vi "Teleop.vi"(10 "Match Info":T1={"Autonomous Elapsed Seconds"=0.0, "TeleOp Elapsed Seconds"=0.0, "Disabled Elapsed Seconds"=0.0, "Visited Autonomous"=FALSE, "Visited TeleOp"=FALSE, "Visited Disabled"=FALSE, "Autonomous Settings"={"Autonomous Style"=enum."Independent", "VI Refnum"=refnum}}, 11 "Call Context":T2) -> ()   [LabVIEW 2016]
doc: "This VI is called for each TeleOp packet received from the DS where the robot is not disabled. It is often used to read from the joysticks and update I/O or to update setpoints for timed control loops. It should complete and return within 20 milliseconds or it may miss DS packets."
uses:
  <vilib>/Rock Robotics/WPI/DriverStation/WPI_DriverStationDerivedRobotMode.ctl
  <vilib>/Rock Robotics/WPI/DriverStation/WPI_DriverStationMatch Info.ctl
  <vilib>/Rock Robotics/WPI/Solenoid/WPI_SolenoidValue.ctl
  <vilib>/Rock Robotics/WPI/Utilities/WPI_GetSetVariantRefNum.vi
  <vilib>/Rock Robotics/Network Tables/NT Write Boolean Array.vi
  <vilib>/Rock Robotics/Network Tables/NT Write Numeric Array.vi
  <vilib>/Rock Robotics/Network Tables/NT Read Boolean.vi
  <vilib>/Rock Robotics/Network Tables/NT Read Number.vi
  <vilib>/Rock Robotics/WPI/Solenoid/WPI_SolenoidSetEnum.vi
  <vilib>/Rock Robotics/Network Tables/NT Write Boolean.vi
  <vilib>/Rock Robotics/WPI/RobotDrive/WPI_RobotDriveArcadeDrive_Standard(NoSaturation).vi
panel:
  out "Sample Slider 0":dbl(slide) scale=0.0..5.0
  out "Sample Boolean 1":bool
  out "Sample Boolean 0":bool
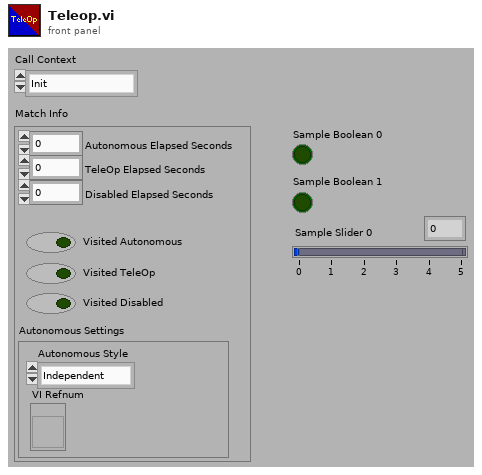
[diagram p1: front panel]
types:
  T1 = typedef "WPI_DriverStationMatch Info.ctl" = cluster{"Autonomous Elapsed Seconds":dbl, "TeleOp Elapsed Seconds":dbl, "Disabled Elapsed Seconds":dbl, "Visited Autonomous":bool, "Visited TeleOp":bool, "Visited Disabled":bool, "Autonomous Settings":cluster{"Autonomous Style":enum16{"Iterative", "Independent"}, "VI Refnum":refnum<vi>}}
  T2 = typedef "WPI_DriverStationDerivedRobotMode.ctl" = enum16{"Init", "Execute", "Stop"}
  T3 = typedef "WPI_SolenoidValue.ctl" = enum16{"Off", "On", "Forward", "Reverse"}
  T4 = typedef "WPI_MotorControlDeviceRef.ctl" = cluster{"DeviceStatus":errorcluster, "Type":T5, "PWM":cluster{"PWM Channel":T6, "DeadBand":T7}, "CAN":cluster{"Device Number":u8, "SetOutput VI Ref":variant, "GetOutput VI Ref":variant, "Enable VI Ref":variant, "Disable VI Ref":variant, "Data":variant}, "Invert":bool}
  T5 = typedef "WPI_MotorControlType.ctl" = enum16{"PWM", "CAN"}
  T6 = typedef "FPGA_DIOPWMChannel.ctl" = enum8{"PWM 0", "PWM 1", "PWM 2", "PWM 3", "PWM 4", "PWM 5", "PWM 6", "PWM 7", "PWM 8", "PWM 9", "PWM MXP 0", "PWM MXP 1", "PWM MXP 2", "PWM MXP 3", "PWM MXP 4", "PWM MXP 5", "PWM MXP 6", "PWM MXP 7", "PWM MXP 8", "PWM MXP 9", "Invalid"}
  T7 = typedef "WPI_PWMDeadband.ctl" = cluster{"Name":string, "maxPositivePwm":i32, "minPositivePwm":i32, "centerPwm":i32, "maxNegativePwm":i32, "minNegativePwm":i32, "angularRange":u16}
  T8 = typedef "WPI_RobotDriveDevRef.ctl" = cluster{"DevStatus":errorcluster, "Motors[]":T4[], "Square Inputs":bool, "Max Output":dbl}
  T9 = typedef "WPI_JoystickDevRef.ctl" = cluster{"Device":T10}
  T10 = typedef "WPI_JoystickDeviceEnum.ctl" = enum16{"USB 0", "USB 1", "USB 2", "USB 3", "USB 4", "USB 5"}
  T11 = typedef "WPI_SolenoidDevRef.ctl" = cluster{"DevStatus":errorcluster, "Pneumatics Control Module":u8, "Forward Solenoid Channel":T12, "Reverse Solenoid Channel":T12}
  T12 = typedef "WPI_SolenoidChannel.ctl" = enum8{"Solenoid 0", "Solenoid 1", "Solenoid 2", "Solenoid 3", "Solenoid 4", "Solenoid 5", "Solenoid 6", "Solenoid 7", "Invalid"}
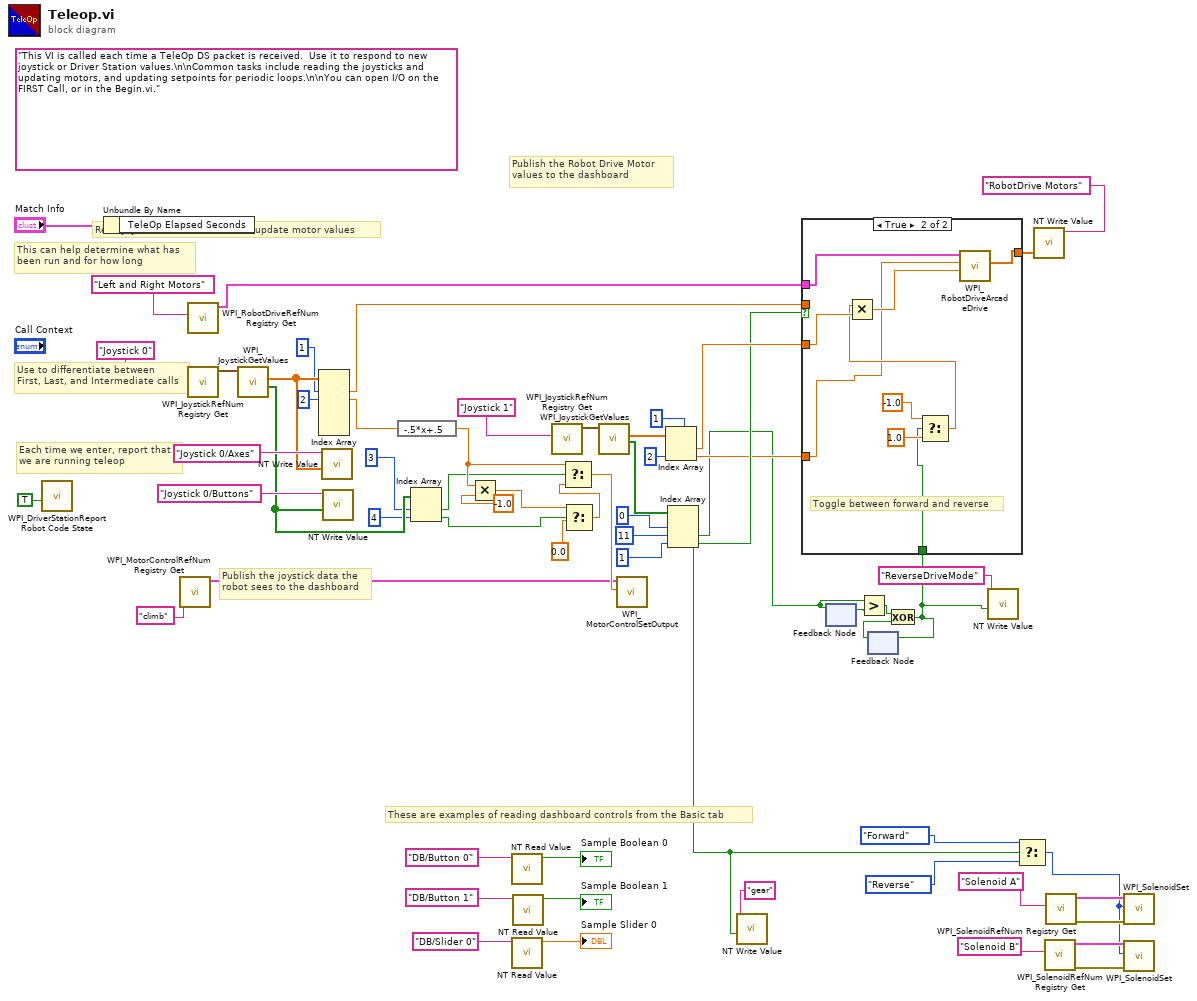
[diagram p0: block diagram]
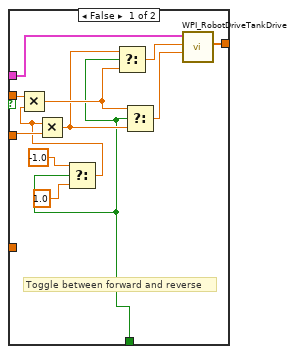
[diagram p2: hidden frame]
diagram:
  (unwired) "This VI is called each time a TeleOp DS packet is received.  Use it to respond to new joystick or Driver Station values.\n\nCommon tasks include reading the joysticks and updating motors, and updating setpoints for periodic loops.\n\nYou can open I/O on the FIRST Call, or in the Begin.vi."
  # "Publish the Robot Drive Motor\nvalues to the dashboard"
  # "These are examples of reading dashboard controls from the Basic tab"
  # "Publish the joystick data the\nrobot sees to the dashboard"
  # "Each time we enter, report that\nwe are running teleop"
  # "Use to differentiate between\nFirst, Last, and Intermediate calls"
  # "This can help determine what has\nbeen run and for how long"
  # "Read Joystick X and Y values and update motor values"
  n1 = call <vilib>:"WPI_DriverStationReport Robot Code State.vi"("TeleOp"=TRUE ("Autonomous")) -> ()  [unwired: 10 in, 1 out]
  n2 = Unbundle By Name("Match Info") -> ()  [unwired: 1 out]
  n3 = call <vilib>:"WPI_MotorControlRefNum Registry Get.vi"("refnum name"="climb") -> ("MotorControlDevRef"=w25:T4)  [unwired: 9 in, 1 out]
  n4 = call <vilib>:"WPI_RobotDriveRefNum Registry Get.vi"("refnum name"="Left and Right Motors") -> ("RobotDriveDevRef"=w20:T8)  [unwired: 1 in, 9 out]
  n5 = call <vilib>:"WPI_JoystickRefNum Registry Get.vi"("refnum name"="Joystick 0") -> ("JoystickDevRef"=w60:T9)  [unwired: 1 in, 9 out]
  n6 = call <vilib>:"WPI_JoystickGetValues.vi"("JoystickDevRef"=w60) -> ("Buttons"=w34:bool[], "Axes"=w56:dbl[])  [unwired: 6 in, 3 out]
  n7 = Index Array(array=w56, index #1=1 ("index"), index #2=2 ("index")) -> (element #1=w19:dbl, element #2=w31:dbl)  [unwired: 4 in, 4 out]
  n8 = call-poly <vilib>:"NT Write Value.vi"("Numeric Array"=w56, "Name"="Joystick 0/Axes") -> ()  [unwired: 9 in, 1 out]
  n9 = call-poly <vilib>:"NT Write Value.vi"("Boolean Array"=w34, "Name"="Joystick 0/Buttons") -> ()  [unwired: 9 in, 1 out]
  n10 = expression code="-.5*x+.5"(w31) -> (w30:dbl)
  n11 = Index Array(array=w34, index #1=3 ("index"), index #2=4 ("index")) -> (element #1=w21:bool, element #2=w22:bool)
  n12 = Multiply(x=w30, y=-1.0) -> (x*y=w27:dbl)
  n13 = call-poly <vilib>:"NT Read Value.vi"("Name"="DB/Button 0" ("refnum name")) -> ("Boolean"=→"Sample Boolean 0":bool)  [unwired: 9 in, 1 out]
  n14 = call-poly <vilib>:"NT Read Value.vi"("Name"="DB/Slider 0" ("refnum name")) -> ("Numeric"=→"Sample Slider 0":dbl)  [unwired: 9 in, 1 out]
  n15 = call-poly <vilib>:"NT Read Value.vi"("Name"="DB/Button 1" ("refnum name")) -> ("Boolean"=→"Sample Boolean 1":bool)  [unwired: 9 in, 1 out]
  n16 = call <vilib>:"WPI_JoystickRefNum Registry Get.vi"("refnum name"="Joystick 1") -> ("JoystickDevRef"=w38:T9)  [unwired: 1 in, 9 out]
  n17 = Select(t=w27, s=w22, f=0.0) -> (s? t:f=w23:dbl)
  n18 = Select(t=w30, s=w21, f=w23) -> (s? t:f=w28:dbl)
  n19 = call <vilib>:"WPI_JoystickGetValues.vi"("JoystickDevRef"=w38) -> ("Buttons"=w11:bool[], "Axes"=w37:dbl[])  [unwired: 6 in, 3 out]
  n20 = call <vilib>:"WPI_MotorControlSetOutput.vi"("Output"=w28, "MotorControlDevRef"=w25) -> ()  [unwired: 7 in, 3 out]
  n21 = Index Array(array=w37, index #1=1 ("index"), index #2=2 ("index")) -> (element #1=w18:dbl, element #2=w13:dbl)
  n22 = Index Array(array=w11, index #1=0 ("index"), index #2=11 ("index"), index #3=1 ("index")) -> (element #1=w8:bool, element #2=w3:bool, element #3=w14:bool)
  n23 = call-poly <vilib>:"NT Write Value.vi"("Boolean"=w8, "Name"="gear") -> ()  [unwired: 9 in, 1 out]
  n24 = feedback #1() -> (w5:bool)  [unwired: 1 in]
  n25 = feedback-in #1(w3) -> ()
  n26 = Greater?(x=w3, y=w5) -> (0:w4:bool)
  n27 = feedback #2() -> (w6:bool)  [unwired: 1 in]
  n28 = Exclusive Or(1:w6, 2:w4) -> (0:w2:bool)
  n29 = case shown="True" w14 {
    tunnel: w20 -> [w70 w83]
    tunnel: w19 -> [w73 _]
    tunnel: w18 -> [w71 w80]
    tunnel: [w72 w84] -> w16
    tunnel: w13 -> [_ w76]
    tunnel: w2 -> [w64 w77]
    frame False {
      # "Toggle between forward and reverse"
      n30 = Select(t=-1.0, s=w64, f=1.0) -> (s? t:f=w65:dbl)
      n31 = Multiply(x=w73, y=w65) -> (x*y=w68:dbl)
      n32 = Multiply(x=w65, y=w71) -> (x*y=w66:dbl)
      n33 = Select(t=w66, s=w64, f=w68) -> (s? t:f=w67:dbl)
      n34 = Select(t=w68, s=w64, f=w66) -> (s? t:f=w69:dbl)
      n35 = call <vilib>:"WPI_RobotDriveTankDrive.vi"("Right axis value"=w69, "Left axis value"=w67, "RobotDriveDevRef"=w70) -> ("Motor Values"=w72:dbl[])  [unwired: 6 in, 2 out]
    }
    frame True {
      # "Toggle between forward and reverse"
      n36 = Select(t=-1.0, s=w77, f=1.0) -> (s? t:f=w79:dbl)
      n37 = Multiply(x=w79, y=w80) -> (x*y=w78:dbl)
      n38 = call-poly <vilib>:"WPI_RobotDriveArcadeDrive.vi"("Y axis value"=w78, "X axis value"=w76, "RobotDriveDevRef"=w83) -> ("Motor Values"=w84:dbl[])  [unwired: 6 in, 2 out]
    }
  }
  n39 = feedback-in #2(w2) -> ()
  n40 = call-poly <vilib>:"NT Write Value.vi"("Boolean"=w2, "Name"="ReverseDriveMode") -> ()  [unwired: 9 in, 1 out]
  n41 = Select(t=WPI_SolenoidValue."Forward" ("Value"), s=w8, f=WPI_SolenoidValue."Reverse" ("Value")) -> (s? t:f=w40:T3)
  n42 = call-poly <vilib>:"NT Write Value.vi"("Numeric Array"=w16, "Name"="RobotDrive Motors") -> ()  [unwired: 9 in, 1 out]
  n43 = call <vilib>:"WPI_SolenoidRefNum Registry Get.vi"("refnum name"="Solenoid B") -> ("error out"=w42:errorcluster, "SolenoidDevRef"=w43:T11)  [unwired: 9 in]
  n44 = call <vilib>:"WPI_SolenoidRefNum Registry Get.vi"("refnum name"="Solenoid A") -> ("error out"=w47:errorcluster, "SolenoidDevRef"=w48:T11)  [unwired: 9 in]
  n45 = call-poly <vilib>:"WPI_SolenoidSet.vi"("error in (no error)"=w47, "Value"=w40, "SolenoidDevRef"=w48) -> ()  [unwired: 7 in, 2 out]
  n46 = call-poly <vilib>:"WPI_SolenoidSet.vi"("error in (no error)"=w42, "Value"=w40, "SolenoidDevRef"=w43) -> ()  [unwired: 7 in, 2 out]
